vi "Read Results from processing.vi"(8 "error in":errorcluster, 11 "ThreePhasePLL runtime in":refnum<class "ThreePhasePLL runtime.lvclass">) -> (0 "error out":errorcluster, 2 "Results from processing":T1, 3 "ThreePhasePLL runtime out":refnum<class "ThreePhasePLL runtime.lvclass">)   [LabVIEW 2017, in "ThreePhasePLL runtime.lvclass"]
uses:
  ThreePhasePLL runtime.lvclass
  configuration/result data indices.ctl
  ThreePhasePLL runtime.lvclass/ThreePhasePLL runtime.ctl
  configuration/ThreePhasePLL configuration.lvclass
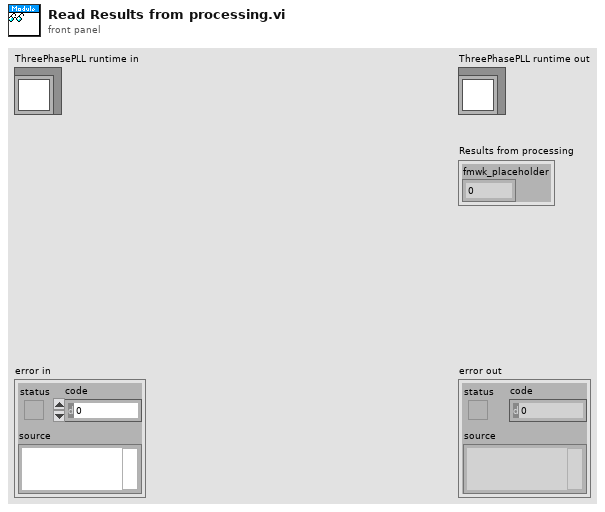
[diagram p1: front panel]
types:
  T1 = typedef "ThreePhasePLL configuration.lvclass/result data indices.ctl" = cluster{"fmwk_placeholder":i32}
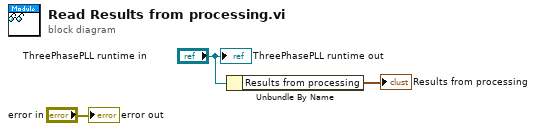
[diagram p0: block diagram]
diagram:
  n1 = Unbundle By Name("ThreePhasePLL runtime in") -> ("Results from processing"=→"Results from processing":T1)
  "error out" <- "error in"
  "ThreePhasePLL runtime out" <- "ThreePhasePLL runtime in"
